vi "Helper Loop Create.vi"(10 "Helper Loop":refnum<class "Helper Loop.lvclass">, 11 "Dev Actor in":refnum<class "Dev Actor.lvclass">) -> (3 "Dev Actor out":refnum<class "Dev Actor.lvclass">)   [LabVIEW 2021, in "Dev Actor.lvlib" / "Dev Actor.lvclass"]
uses:
  Dev Actor.lvclass
  Dev Actor.lvclass/Dev Actor.ctl
  Helper Loop/Helper Loop/Helper Loop.lvclass
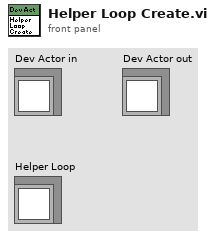
[diagram p1: front panel]
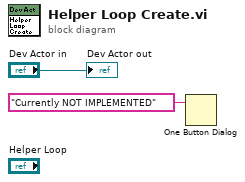
[diagram p0: block diagram]
diagram:
  n1 = One Button Dialog(message="Currently NOT IMPLEMENTED") -> ()  [unwired: 1 in, 1 out]
  "Dev Actor out" <- "Dev Actor in"
